vi "Fetch Run Start Times.vi"(0 "Queue in":refnum<queue>, 5 "Analytics Refs":T1, 7 "Old Value":T2, 9 "New Value":T2, 11 "error in (no error)":errorcluster) -> (4 "Queue out":refnum<queue>, 6 "Start Run Times":string[][](array[string]), 8 "Serial Numbers":string[](array[string]), 10 "Date":string, 14 "Serial Number Header?":bool, 15 "error out":errorcluster)   [LabVIEW 2026, in "Analysis.lvlib"]
uses:
  Analysis.lvlib
  support/Architecture/Message Queue/Message Cluster.ctl
  Test Results.ctl
  Test Details.ctl
  controls/UI/Analytics Refs.ctl
  controls/Messaging Payloads/MSG FetchSensorID Payload.ctl
  controls/UI/UI List Type.ctl
  Database/Database.lvlib
  Settings/Settings.lvlib
  support/Architecture/Message Queue/Message Queue.lvlib
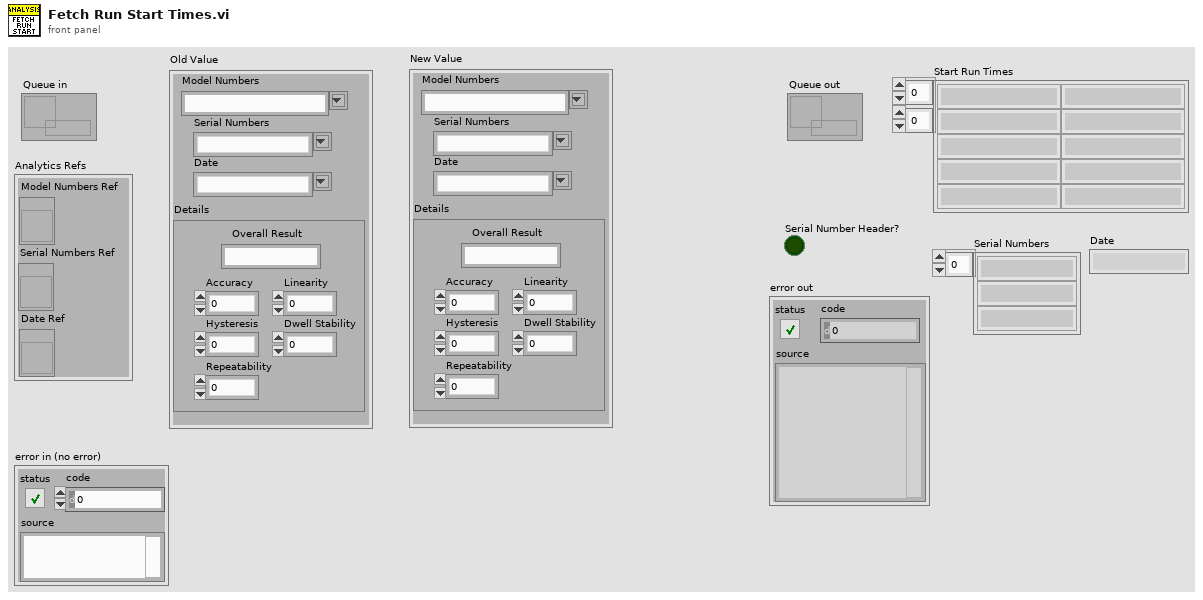
[diagram p1: front panel]
types:
  T1 = typedef "Analysis.lvlib/Analytics Refs.ctl" = cluster{"Model Numbers Ref":refnum<vi>, "Serial Numbers Ref":refnum<vi>, "Date Ref":refnum<vi>}
  T2 = typedef "Analysis.lvlib/Test Results.ctl" = cluster{"Model Numbers":string, "Serial Numbers":string, "Date":string, "Details":T3}
  T3 = typedef "Analysis.lvlib/Test Details.ctl" = cluster{"Accuracy":dbl, "Hysteresis":dbl, "Repeatability":dbl, "Linearity":dbl, "Dwell Stability":dbl, "Overall Result":string}
  T4 = enum8{"Enabled", "Disabled", "Disabled and Grayed Out"}
  T5 = typedef "UI List Type.ctl" = enum16{"Model Numbers", "Serial Numbers", "Operators", "Calibration Points", "Start Run Times"}
  T6 = typedef "Database.lvlib/MSG FetchSensorID Payload.ctl" = cluster{"SensorID":i32, "Serial Number":string, "Model Number":string}
  T7 = typedef "MSG FetchConfiguration Payload.ctl" = cluster{"Serial Numbers":string[], "Hardware Settings Cluster":T8}
  T8 = typedef "Acquisition.lvlib/Instrument Specifications Cluster Configuration.ctl" = cluster{"Sensor ID":i32, "Target Sample Rate (Hz)":dbl, "Steady-State Duration (s)":i32, "Allowed Tolerance (%)":dbl, "Max Settling Timeout (s)":i32, "Physical Channel":string, "Measurement Role":T9}
  T9 = typedef "Settings.lvlib/Measurement Role.ctl" = enum16{"Controller", "Reference", "UUT", "Disable", "All"}
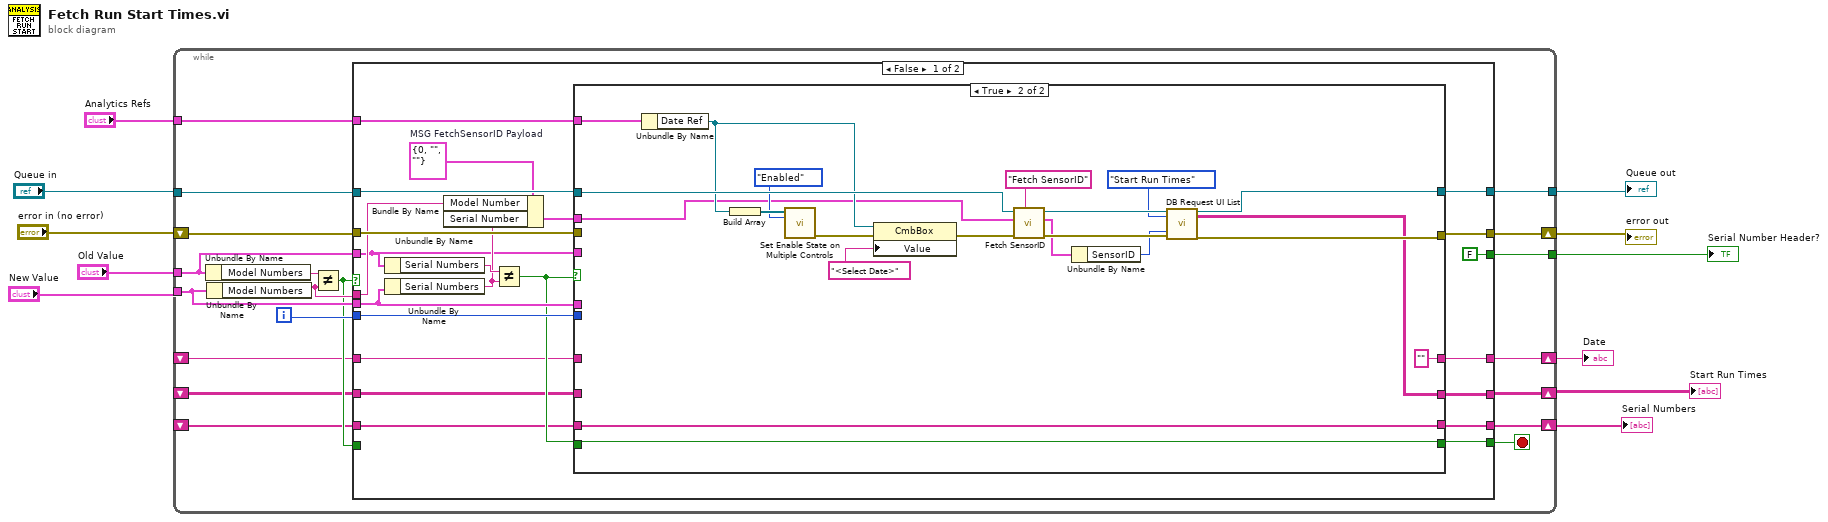
[diagram p0: block diagram]
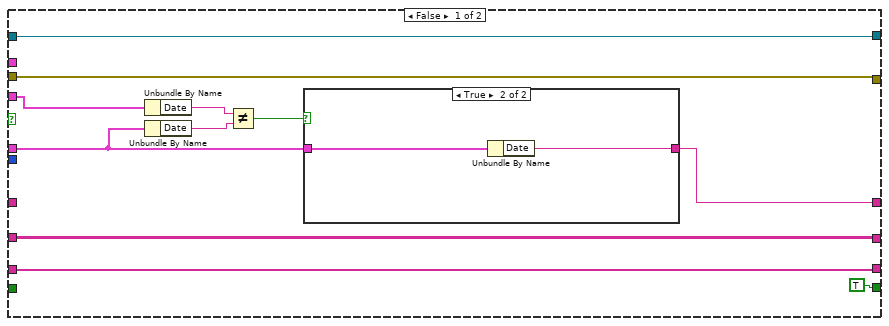
[diagram p2: hidden frame]
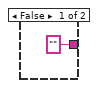
[diagram p3: hidden frame]
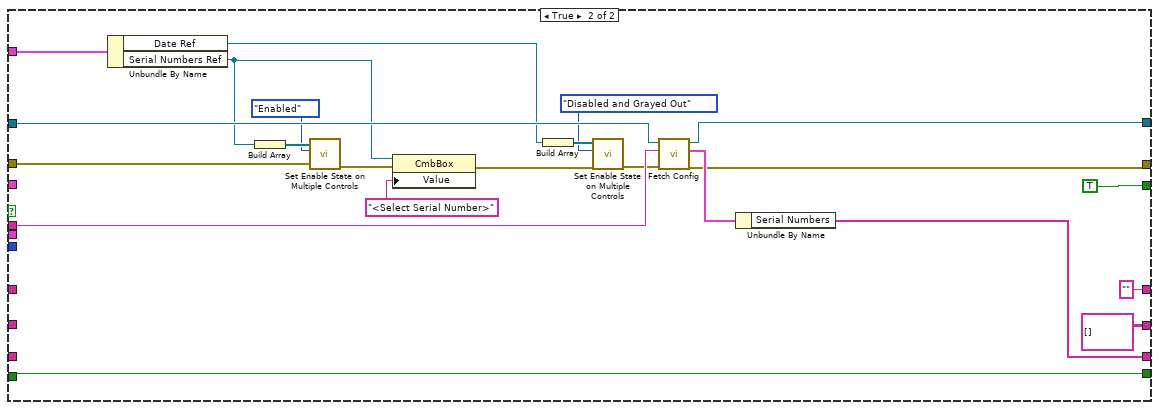
[diagram p4: hidden frame]
diagram:
  n1 = while {
    tunnel: "Old Value" -> [w28]
    tunnel: "New Value" -> [w23]
    tunnel: "Queue in" -> [w30]
    shift-right: [w27] -> w9
    shift-left: "error in (no error)" -> [w26]
    tunnel: [w25] -> w11
    tunnel: [w21] -> w7
    shift-right: [w18] -> w4
    shift-left: _ -> [w16]
    shift-right: [w17] -> w3
    shift-left: _ -> [w15]
    shift-right: [w14] -> w2
    shift-left: _ -> [w13]
    tunnel: "Analytics Refs" -> [w12]
    i -> [w24]
    stop <- w19 stop-if-true
    n2 = Unbundle By Name(w28) -> ("Model Numbers"=w29:string)
    n3 = Unbundle By Name(w23) -> ("Model Numbers"=w22:string)
    n4 = Not Equal?(x=w29, y=w22) -> (x != y?=w20:bool)
    n5 = case shown="False" w20 {
      tunnel: w30 -> [w51 w109]
      tunnel: w28 -> [w42 _]
      tunnel: w26 -> [w50 w94]
      tunnel: [w47 w105] -> w27
      tunnel: [w49 w107] -> w25
      tunnel: w24 -> [w48 _]
      tunnel: w23 -> [w41 _]
      tunnel: w22 -> [w44 w106]
      tunnel: [FALSE TRUE] -> w21
      tunnel: [w39 w103] -> w19
      tunnel: w20 -> [_ w103]
      tunnel: [w37 string[][] [] ("Results")] -> w18
      tunnel: [w34 w102] -> w17
      tunnel: w16 -> [w36 _]
      tunnel: w15 -> [w35 _]
      tunnel: [w33 "" ("Date")] -> w14
      tunnel: w13 -> [w32 _]
      tunnel: w12 -> [w31 w99]
      frame False {
        w46 = T6 {"SensorID"=0, "Serial Number"="", "Model Number"=""}  # MSG FetchSensorID Payload
        n6 = Unbundle By Name(w42) -> ("Serial Numbers"=w52:string)
        n7 = Unbundle By Name(w41) -> ("Serial Numbers"=w43:string)
        n8 = Bundle By Name(cluster=w46, "Model Number"=w44, "Serial Number"=w43) -> (w45:T6)
        n9 = Not Equal?(x=w52, y=w43) -> (x != y?=w38:bool)
        n10 = case shown="True" w38 {
          tunnel: w51 -> [w62 w87]
          tunnel: w50 -> [w63 _]
          tunnel: [w63 w82] -> w47
          tunnel: [w62 w81] -> w49
          tunnel: w48 -> [_ _]
          tunnel: w45 -> [_ w68]
          tunnel: w42 -> [w55 _]
          tunnel: w41 -> [w54 _]
          tunnel: w38 -> [_ w85]
          tunnel: [TRUE w85] -> w39
          tunnel: [w60 w77] -> w37
          tunnel: w36 -> [w60 _]
          tunnel: w35 -> [w59 w76]
          tunnel: [w59 w76] -> w34
          tunnel: [w58 "" ("Date")] -> w33
          tunnel: w32 -> [_ _]
          tunnel: w31 -> [_ w73]
          frame False {
            n11 = Unbundle By Name(w55) -> ("Date"=w57:string)
            n12 = Unbundle By Name(w54) -> ("Date"=w56:string)
            n13 = Not Equal?(x=w57, y=w56) -> (x != y?=w53:bool)
            n14 = case shown="True" w53 {
              tunnel: w54 -> [_ w66]
              tunnel: ["" ("Date") w65] -> w58
              frame False {
              }
              frame True {
                n15 = Unbundle By Name(w66) -> ("Date"=w65:string)
              }
            }
          }
          frame True {
            n16 = Unbundle By Name(w73) -> ("Date Ref"=w70:refnum<vi>)
            n17 = Build Array(w70) -> (w75:refnum<vi>[])
            n18 = call "Set Enable State on Multiple Controls.vi"("Controls"=w75, "Disabled"=T4."Enabled") -> ("error out"=w71:errorcluster)  [unwired: 8 in]
            n19 = property class="CmbBox"(reference=w70, error in=w71, "Value"="<Select Date>") -> (error out=w69:errorcluster)  [unwired: 1 out]
            n20 = call "Fetch SensorID.vi"("Message"="Fetch SensorID", "error in (no error)"=w69, "MSG FetchSensorID Payload in"=w68, "Database in"=w87) -> ("error out"=w83:errorcluster, "MSG FetchSensorID Payload out"=w80:T6, "Database out"=w84:refnum<queue>)  [unwired: 5 in]
            n21 = Unbundle By Name(w80) -> ("SensorID"=w78:i32)
            n22 = call "DB Request UI List.vi"("Database in"=w84, "UI List Type"=UI_List_Type."Start Run Times", "Identifier"=w78, "error in (no error)"=w83) -> ("Database out"=w81:refnum<queue>, "Results"=w77:string[][], "error out"=w82:errorcluster)  [unwired: 13 in]
          }
        }
      }
      frame True {
        n23 = Unbundle By Name(w99) -> ("Date Ref"=w92:refnum<vi>, "Serial Numbers Ref"=w88:refnum<vi>)
        n24 = Build Array(w88) -> (w98:refnum<vi>[])
        n25 = call "Set Enable State on Multiple Controls.vi"("Controls"=w98, "Disabled"=T4."Enabled", "error in (no error)"=w94) -> ("error out"=w90:errorcluster)  [unwired: 7 in]
        n26 = property class="CmbBox"(reference=w88, error in=w90, "Value"="<Select Serial Number>") -> (error out=w89:errorcluster)  [unwired: 1 out]
        n27 = Build Array(w92) -> (w96:refnum<vi>[])
        n28 = call "Set Enable State on Multiple Controls.vi"("Controls"=w96, "Disabled"=T4."Disabled and Grayed Out", "error in (no error)"=w89) -> ("error out"=w93:errorcluster)  [unwired: 7 in]
        n29 = call "Fetch Config.vi"("error in (no error)"=w93, "ModelNumber"=w106, "Database in"=w109) -> ("error out"=w105:errorcluster, "Model Details Payload"=w108:T7, "Database out"=w107:refnum<queue>)  [unwired: 6 in]
        n30 = Unbundle By Name(w108) -> ("Serial Numbers"=w102:string[])
      }
    }
  }
  "Queue out" <- w11
  "error out" <- w9
  "Serial Number Header?" <- w7
  "Start Run Times" <- w4
  "Serial Numbers" <- w3
  "Date" <- w2
